vi "DSF Transfer Group.Set Current Iteration.vi"(8 "error in (no error)":errorcluster, 10 "iteration":u64=1, 11 "Transfer Group in":refnum<class "Transfer Group.lvclass">) -> (0 "error out":errorcluster, 3 "Transfer Group out":refnum<class "Transfer Group.lvclass">)   [LabVIEW 2017, in "DSF Core.lvlib" / "Transfer Group.lvclass"]
uses:
  Transfer Group.lvclass
  Transfer Group.lvclass/Transfer Group.ctl
  Timing/Timing.lvclass/Timing.ctl
  Timing/Timing.Set Iteration.vi
  Timing/Timing.lvclass
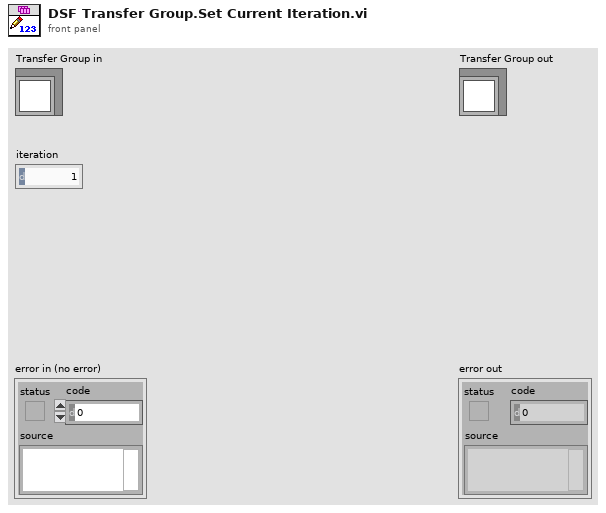
[diagram p1: front panel]
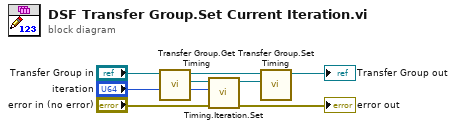
[diagram p0: block diagram]
diagram:
  n1 = call "Transfer Group.Get Timing.vi"("Transfer Group in"="Transfer Group in") -> ("Timing"=w7:refnum<class "Timing.lvclass">, "Transfer Group out"=w3:refnum<class "Transfer Group.lvclass">)  [unwired: 9 in]
  n2 = call "Timing.Iteration.Set.vi"("error in (no error)"="error in (no error)", "iteration"="iteration", "Timing in"=w7) -> ("error out"=→"error out":errorcluster, "Timing out"=w4:refnum<class "Timing.lvclass">)  [unwired: 7 in]
  n3 = call "Transfer Group.Set Timing.vi"("Timing"=w4, "Transfer Group in"=w3) -> ("Transfer Group out"=→"Transfer Group out":refnum<class "Transfer Group.lvclass">)  [unwired: 9 in]
